vi "test_TrajectoryCN090716SpiralScan.vi"() -> ()   [LabVIEW 2010, in "TrajectoryCN090716SpiralScan.lvclass"]
uses:
  TrajectoryCN090716SpiralScan.lvclass
  <vilib>/Native 3D Graph/xcontrol/3DPC_SurfacePlot.xctl
  common/enumerations/x_y_z_enumeration.ctl
  common/enumerations/functional_global_action_enum.ctl
panel:
  in  "repetition rate":dbl[unit]=10.0
  out "z uncorrected":dbl[](graph)
  in  "defineButton":bool
  in  "analyseButton":bool
  out "XY projection":cluster{"Y":dbl[], "Y":dbl[]}[](graph)
  out "combined x,y,z plots":dbl[][](graph)
  out "3D Graph":refnum<class "Base Datatype.lvclass">[](xcontrol)
  in  "stop":bool
  # "Test TrajectoryCN090716SpiralScan"
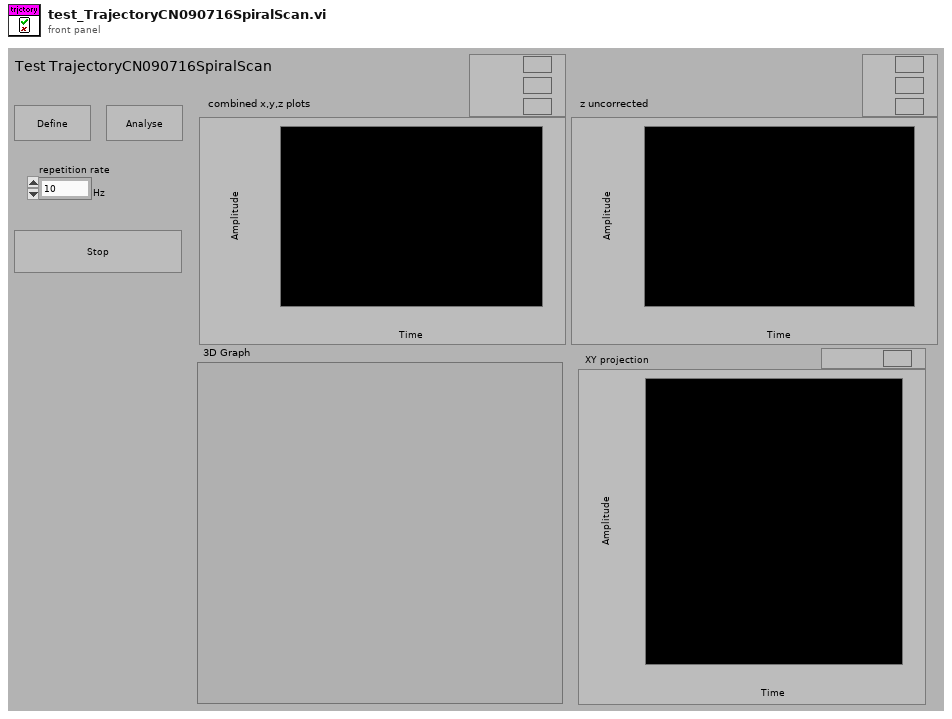
[diagram p1: front panel]
types:
  T1 = typedef "x_y_z_enumeration.ctl" = enum16{"x", "y", "z"}
  T2 = typedef "functional_global_action_enum.ctl" = enum16{"get", "set", "reset"}
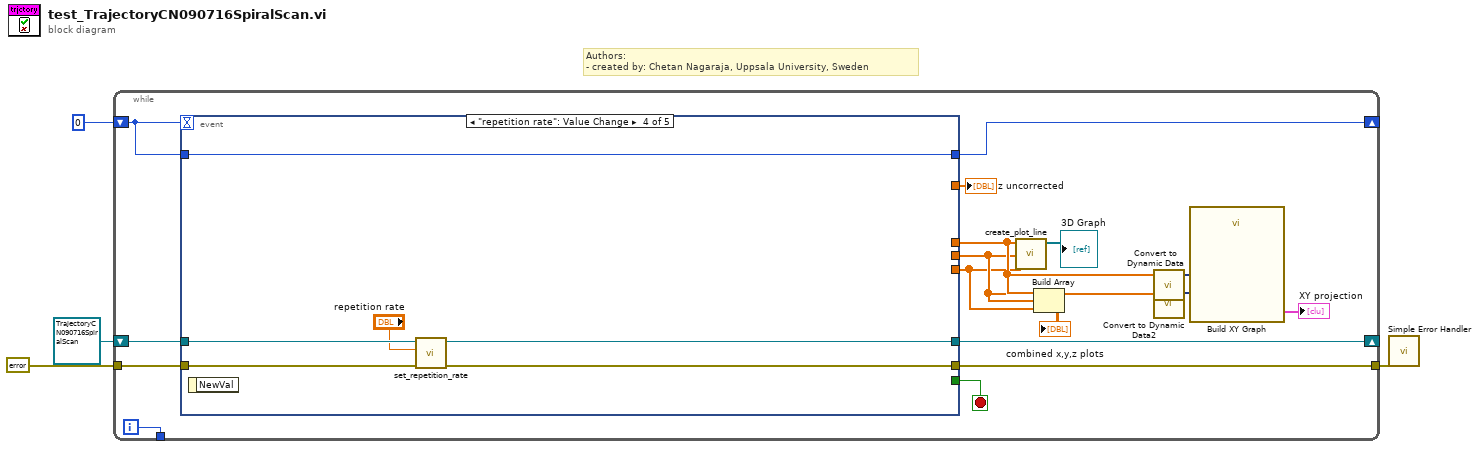
[diagram p0: block diagram]
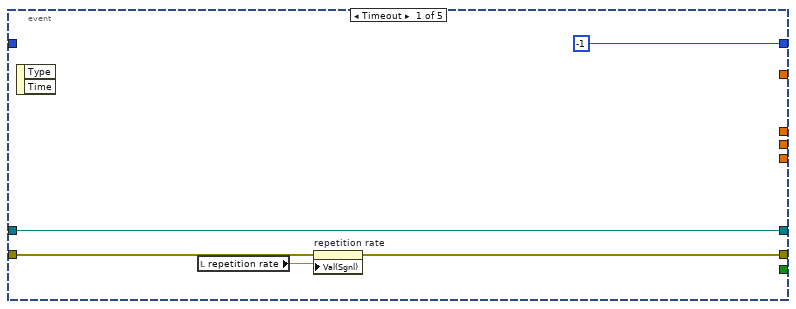
[diagram p2: hidden frame]
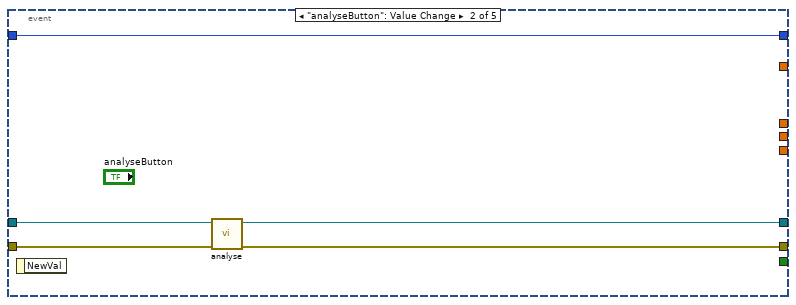
[diagram p3: hidden frame]
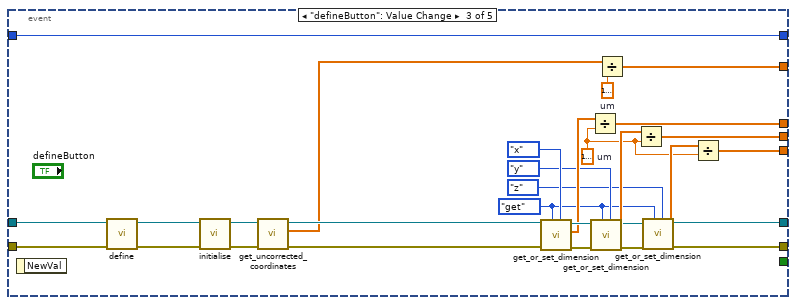
[diagram p4: hidden frame]
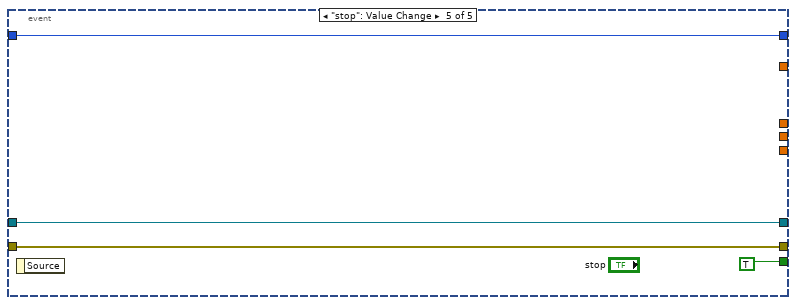
[diagram p5: hidden frame]
diagram:
  # "Authors: \n- created by: Chetan Nagaraja, Uppsala University, Sweden"
  n1 = while {
    shift-right: [w16] -> _
    shift-left: 0 -> [w21]
    tunnel: errorcluster {"status"=FALSE, "code"=0, "source"=""} ("error in (no error)") -> [w19]
    shift-right: [w14] -> _
    shift-left: refnum<class "TrajectoryCN090716SpiralScan.lvclass"> refnum ("TrajectoryCN090716SpiralScan.lvclass") -> [w20]
    tunnel: [w18] -> _
    tunnel: [w15] -> w1
    i -> [w18]
    stop <- w17 stop-if-true
    n2 = event shown="[3] \"repetition rate\": Value Change" {
      selector: _ -> [_ _ _ _ _]
      dyn-events: _ -> [_ _ _ _ _]
      timeout: w21 -> [_ _ _ _ _]
      tunnel: [-1 w31 w60 w66 w70] -> w16
      tunnel: w21 -> [_ w31 w60 w66 w70]
      tunnel: w20 -> [w26 w30 w58 w63 w69]
      tunnel: [w26 w27 w42 w62 w69] -> w14
      tunnel: [w23 w29 w44 w64 w68] -> w15
      tunnel: w19 -> [w24 w28 w59 w65 w68]
      tunnel: [_ _ _ _ TRUE] -> w17
      tunnel: [_ _ w41 _ _] -> w8
      tunnel: [_ _ w35 _ _] -> w10
      tunnel: [_ _ w40 _ _] -> w6
      tunnel: [_ _ w34 _ _] -> w5
      event Timeout {
        n3 = event-data() -> ()  [unwired: 3 out]
        n4 = local read "repetition rate"() -> (w22:dbl[unit])
        n5 = property on="repetition rate" class="DigNum (strict)"(error in=w24, "Val(Sgnl)"=w22) -> (error out=w23:errorcluster)  [unwired: 1 in, 1 out]
      }
      event "analyseButton": Value Change {
        n6 = event-data() -> ()  [unwired: 2 out]
        n7 = call-dynamic "analyse.vi"("error in (no error)"=w28, "TrajectoryDL091126GenericVoxel in"=w30) -> ("error out"=w29:errorcluster, "TrajectoryDL091126GenericVoxel out"=w27:refnum<class "TrajectoryCN090716SpiralScan.lvclass">)  [unwired: 8 in]
      }
      event "defineButton": Value Change {
        w33 = dbl[unit] 1e-06  # um
        w46 = dbl[unit] 1e-06  # um
        w51 = functional_global_action_enum."get" ("action")
        n8 = event-data() -> ()  [unwired: 2 out]
        n9 = call-dynamic "define.vi"("error in (no error)"=w59, "TrajectoryCN090716SpiralScan in"=w58) -> ("error out"=w45:errorcluster, "TrajectoryCN090716SpiralScan out"=w43:refnum<class "TrajectoryCN090716SpiralScan.lvclass">)  [unwired: 8 in]
        n10 = call-dynamic "initialise.vi"("error in (no error)"=w45, "TrajectoryCN090716SpiralScan in"=w43) -> ("error out"=w39:errorcluster, "TrajectoryCN090716SpiralScan out"=w38:refnum<class "TrajectoryCN090716SpiralScan.lvclass">)  [unwired: 8 in]
        n11 = call-dynamic "get_uncorrected_coordinates.vi"("error in (no error)"=w39, "TrajectoryCN090716SpiralScan in"=w38) -> ("error out"=w36:errorcluster, "z"=w32:dbl[unit][], "TrajectoryCN090716SpiralScan out"=w37:refnum<class "TrajectoryCN090716SpiralScan.lvclass">)  [unwired: 5 in, 2 out]
        n12 = call-dynamic "get_or_set_dimension.vi"("dimension"=x_y_z_enumeration."x", "action"=w51, "error in (no error)"=w36, "GenericTrajectory in"=w37) -> ("error out"=w56:errorcluster, "pixel values out (single dimension)"=w54:dbl[unit][], "GenericTrajectory out"=w57:refnum<class "TrajectoryCN090716SpiralScan.lvclass">)  [unwired: 2 in, 3 out]
        n13 = Divide(x=w54, y=w46) -> (x/y=w35:dbl[])
        n14 = call-dynamic "get_or_set_dimension.vi"("dimension"=x_y_z_enumeration."y", "action"=w51, "error in (no error)"=w56, "GenericTrajectory in"=w57) -> ("error out"=w48:errorcluster, "pixel values out (single dimension)"=w53:dbl[unit][], "GenericTrajectory out"=w49:refnum<class "TrajectoryCN090716SpiralScan.lvclass">)  [unwired: 2 in, 3 out]
        n15 = Divide(x=w32, y=w33) -> (x/y=w34:dbl[])
        n16 = Divide(x=w53, y=w46) -> (x/y=w41:dbl[])
        n17 = call-dynamic "get_or_set_dimension.vi"("dimension"=x_y_z_enumeration."z", "action"=w51, "error in (no error)"=w48, "GenericTrajectory in"=w49) -> ("error out"=w44:errorcluster, "pixel values out (single dimension)"=w47:dbl[unit][], "GenericTrajectory out"=w42:refnum<class "TrajectoryCN090716SpiralScan.lvclass">)  [unwired: 5 in]
        n18 = Divide(x=w47, y=w46) -> (x/y=w40:dbl[])
      }
      event "repetition rate": Value Change {
        n19 = event-data() -> ()  [unwired: 2 out]
        n20 = call-dynamic "set_repetition_rate.vi"("error in (no error)"=w65, "repetition rate"="repetition rate", "GenericTrajectory in"=w63) -> ("error out"=w64:errorcluster, "GenericTrajectory out"=w62:refnum<class "TrajectoryCN090716SpiralScan.lvclass">)  [unwired: 7 in]
      }
      event "stop": Value Change {
        n21 = event-data() -> ()  [unwired: 2 out]
      }
    }
    "z uncorrected" <- w5
    n22 = call <vilib>:"create_plot_line.vi"("z vector"=w6, "y vector"=w8, "x vector"=w10) -> ("plots out"=→"3D Graph":refnum<class "Base Datatype.lvclass">[])  [unwired: 2 in, 6 out]
    n23 = Build Array(w10, w8, w6) -> (→"combined x,y,z plots":dbl[][])
    n24 = call "Convert to Dynamic Data"("Array"=w10) -> ("Dynamic Data Type"=w9:dynamicdata)  [unwired: 3 in]
    n25 = call "Convert to Dynamic Data2"("Array"=w8) -> ("Dynamic Data Type"=w7:dynamicdata)  [unwired: 3 in]
    n26 = call "Build XY Graph"("Y Input"=w7, "X Input"=w9) -> ("XY Graph"=→"XY projection":cluster{"Y":dbl[], "Y":dbl[]}[])  [unwired: 8 in, 1 out]
  }
  n27 = call <vilib>:"Simple Error Handler.vi"("error in (no error)"=w1) -> ()  [unwired: 1 in, 8 out]
